vi "Populate SCL v2.vi"(8 "error in":errorcluster, 11 "SCL":refnum<vi>) -> (0 "error out":errorcluster, 3 "At least one template file found?":bool)   [LabVIEW 2020]
doc: "Populates the two SCLs that display the available VI templates and CTL templates, respectively.\n\nSCL = Single-Column Listbox"
uses:
  <vilib>/Utility/miscctls.llb/LVFontTypeDef.ctl
panel:
  out "All Template Filenames":string[](array[string])
  out "CTTs":string[](array[string])
  out "VITs":string[](array[string])
  out "VIs":string[](array[string])
  out "CTLs":string[](array[string])
  out "Templates Folder Location":path
  out "All Filenames In Folder":string[](array[string])
  # "Development\ncontrols/indicators useful for development and testing, but which are not outputs of the VI"
  # "Input\nInputs to the VI"
  # "Output\nOutputs of the VI"
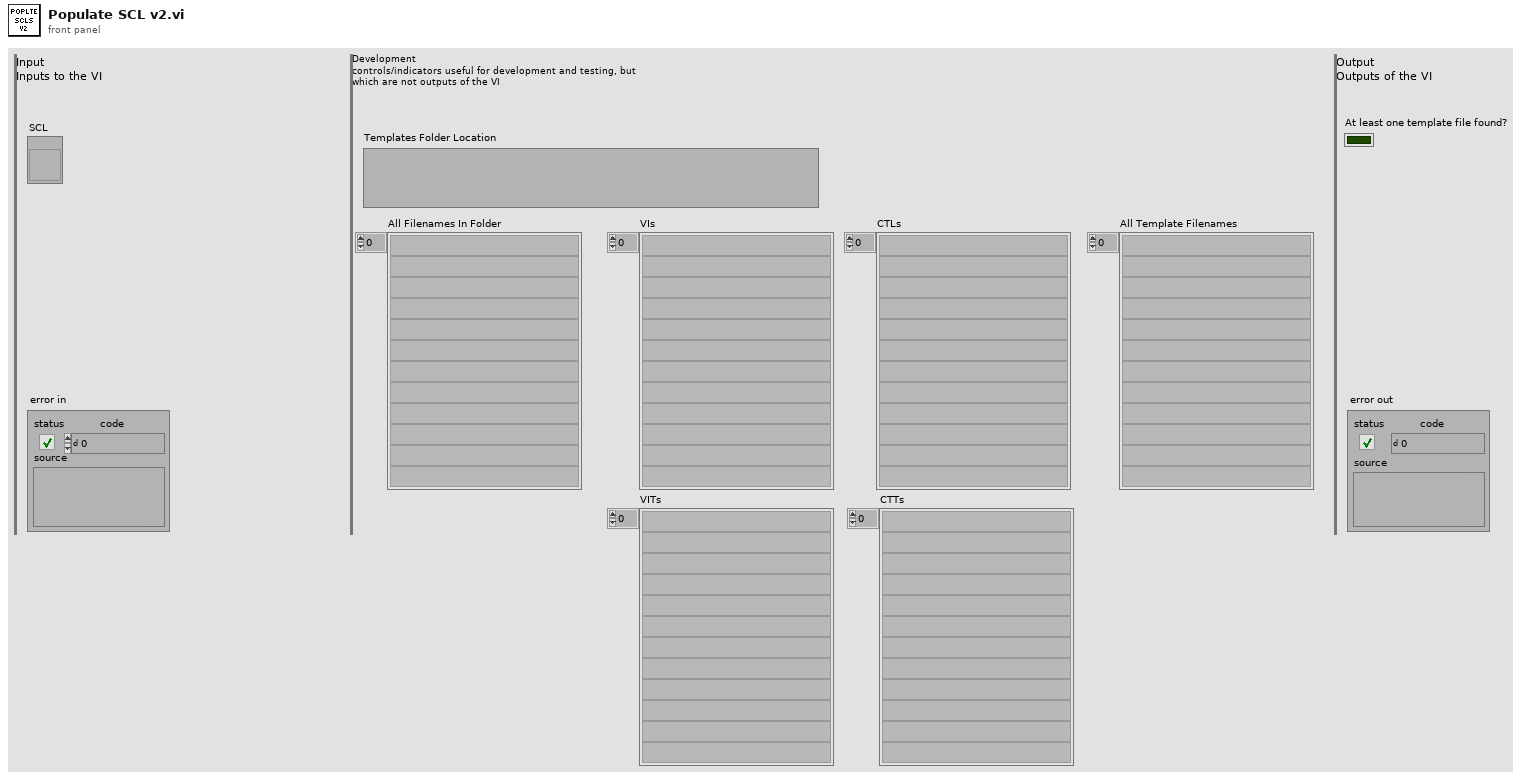
[diagram p1: front panel]
types:
  T1 = typedef "LVFontTypeDef.ctl" = cluster{"Font Name":string, "Size":u16, "Bold":bool, "Italic":bool, "Underline":bool, "Strikeout":bool, "Color":u32}
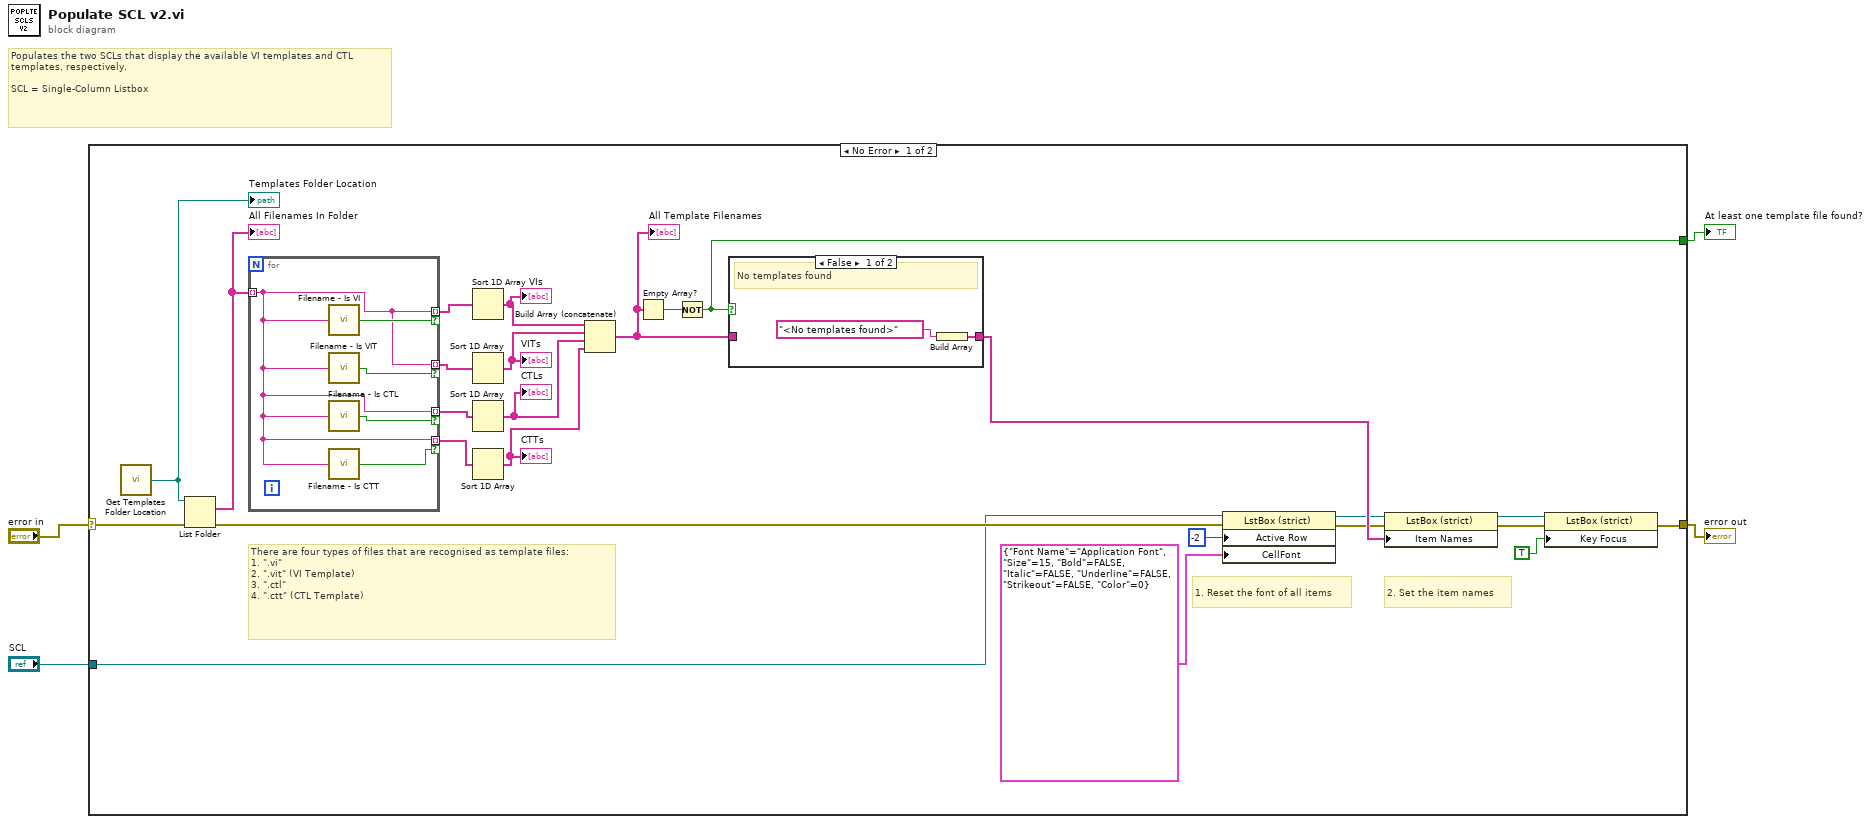
[diagram p0: block diagram]
diagram:
  # "Populates the two SCLs that display the available VI templates and CTL templates, respectively.\n\nSCL = Single-Column Listbox"
  n1 = case shown="No Error" "error in" {
    selector: "error in" -> [w29 w38]
    tunnel: [w21 w38] -> w3
    tunnel: "SCL" -> [w25 _]
    tunnel: [w5 _] -> w1
    frame No Error {
      # "2. Set the item names"
      # "1. Reset the font of all items"
      # "There are four types of files that are recognised as template files:\n1. \".vi\"\n2. \".vit\" (VI Template)\n3. \".ctl\"\n4. \".ctt\" (CTL Template)"
      n2 = call "Get Templates Folder Location.vi"() -> ("Templates Folder Location"=w22:path)
      "Templates Folder Location" <- w22
      n3 = List Folder(path=w22, error in=w29) -> (filenames=w27:string[], error out=w28:errorcluster)  [unwired: 2 in, 2 out]
      "All Filenames In Folder" <- w27
      n4 = for {
        tunnel: w27 -> [w34] mode=indexing
        tunnel: [w34] -> w26 mode=indexing if=w37
        tunnel: [w34] -> w18 mode=indexing if=w36
        tunnel: [w34] -> w17 mode=indexing if=w35
        tunnel: [w34] -> w16 mode=indexing if=w33
        n5 = call "Filename - Is VI.vi"("Filename (including file extension)"=w34) -> ("Is VI?"=w37:bool)
        n6 = call "Filename - Is VIT.vi"("Filename (including file extension)"=w34) -> ("Is VIT?"=w36:bool)
        n7 = call "Filename - Is CTL.vi"("Filename (including file extension)"=w34) -> ("Is CTL?"=w35:bool)
        n8 = call "Filename - Is CTT.vi"("Filename (including file extension)"=w34) -> ("Is CTT?"=w33:bool)
      }
      n9 = Sort 1D Array(array=w26) -> (sorted array=w15:string[])
      "VIs" <- w15
      n10 = Sort 1D Array(array=w18) -> (sorted array=w14:string[])
      "VITs" <- w14
      n11 = Sort 1D Array(array=w17) -> (sorted array=w13:string[])
      "CTLs" <- w13
      n12 = Sort 1D Array(array=w16) -> (sorted array=w12:string[])
      "CTTs" <- w12
      n13 = Build Array (concatenate)(w15, w14, w13, w12) -> (w6:string[])
      "All Template Filenames" <- w6
      n14 = Empty Array?(array=w6) -> (empty?=w24:bool)
      n15 = Not(x=w24) -> (.not. x?=w5:bool)
      n16 = case shown="False" w5 {
        tunnel: w6 -> [_ w32]
        tunnel: [w30 w32] -> w11
        frame False {
          # "No templates found"
          n17 = Build Array("<No templates found>") -> (w30:string[])
        }
        frame True {
          # "One or more template files found"
        }
      }
      n18 = property class="LstBox (strict)"(reference=w25, error in=w28, "Active Row"=-2 ("Active Row:Active Row Number"), "CellFont"=T1 {"Font Name"="Application Font", "Size"=15, "Bold"=FALSE, "Italic"=FALSE, "Underline"=FALSE, "Strikeout"=FALSE, "Color"=0} ("Active Row:Cell Font")) -> (reference out=w9:refnum<vi>, error out=w8:errorcluster)
      n19 = property class="LstBox (strict)"(reference=w9, error in=w8, "Item Names"=w11) -> (reference out=w20:refnum<vi>, error out=w23:errorcluster)
      n20 = property class="LstBox (strict)"(reference=w20, error in=w23, "Key Focus"=TRUE) -> (error out=w21:errorcluster)  [unwired: 1 out]
    }
    frame Error {
    }
  }
  "error out" <- w3
  "At least one template file found?" <- w1
